vi "CENTRIOD DETECTION.vi"(0 "Refnum in":T6=refnum, 1 "auto threshold":bool, 2 "Threshold Range In":cluster{"Lower value":sgl, "Upper value":sgl}={"Lower value"=128.0, "Upper value"=255.0} {"Upper value" format="%.2f"; "Lower value" format="%.2f"}, 4 "beam detection para":T4={"Filter"=1, "Filter Para"={"X Size"=5, "Y Size"=5, "% Tolerance"=1}, "detection method"=4, "smal para"=[{"Measurement Parameter"=35, "Range Lower Value"=0.0, "Range Upper Value"=500.0, "Range"=TRUE, "Measurement Type"=FALSE}], "Remove small Objects"=TRUE, "Restrict to round Objects"=TRUE} {"smal para"."Measurement Parameter" items=["Center of Mass X", "Center of Mass Y", "First Pixel X", "First Pixel Y", "Bounding Rect Left", "Bounding Rect Top", "Bounding Rect Right", "Bounding Rect Bottom", "Max Feret Diameter Start X", "Max Feret Diameter Start Y", "Max Feret Diameter End X", "Max Feret Diameter End Y", "Max Horiz. Segment Length Left", "Max Horiz. Segment Length Right", "Max Horiz. Segment Length Row", "-", "Bounding Rect Width", "Bounding Rect Height", "Bounding Rect Diagonal", "Perimeter", "Convex Hull Perimeter", "Holes' Perimeter", "Max Feret Diameter", "Equivalent Ellipse Major Axis", "Equivalent Ellipse Minor Axis", "Equivalent Ellipse Minor Axis (Feret)", "Equivalent Rect Long Side", "Equivalent Rect Short Side", "Equivalent Rect Diagonal", "Equivalent Rect Short Side (Feret)", "Average Horiz. Segment Length", "Average Vert. Segment Length", "Hydraulic Radius", "Waddel Disk Diameter", "-", "Area", "Holes' Area", "Particle & Holes' Area", "Convex Hull Area", "Image Area", "-", "Number of Holes", "Number of Horiz. Segments", "Number of Vert. Segments", "-", "Orientation", "Max Feret Diameter Orientation", "-", "% Area/Image Area", "% Area/(Particle & Holes' Area)", "Ratio of Equivalent Ellipse Axes", "Ratio of Equivalent Rect Sides", "-", "Elongation Factor", "Compactness Factor", "Heywood Circularity Factor", "Type Factor", "-", "Sum X", "Sum Y", "Sum XX", "Sum XY", "Sum YY", "Sum XXX", "Sum XXY", "Sum XYY", "Sum YYY", "-", "Moment of Inertia XX", "Moment of Inertia XY", "Moment of Inertia YY", "Moment of Inertia XXX", "Moment of Inertia XXY", "Moment of Inertia XYY", "Moment of Inertia YYY", "Norm. Moment of Inertia XX", "Norm. Moment of Inertia XY", "Norm. Moment of Inertia YY", "Norm. Moment of Inertia XXX", "Norm. Moment of Inertia XXY", "Norm. Moment of Inertia XYY", "Norm. Moment of Inertia YYY", "Hu Moment 1", "Hu Moment 2", "Hu Moment 3", "Hu Moment 4", "Hu Moment 5", "Hu Moment 6", "Hu Moment 7"]; "smal para"."Range Lower Value" format="%.2f"; "smal para"."Range Upper Value" format="%.2f"; "detection method" items=["clustering", "entropy", "metric", "moments", "inter-class variance"]; "Filter" items=["No Filter", "Median Filter", "Low Pass Filter"]}, 5 "error in (no error)":errorcluster) -> (8 "Bounding Rect":T7={"Left"=200.0, "Top"=222.0, "Right"=337.0, "Bottom"=354.0}, 11 "Particle Reports (Pixels)":T8(array[cluster])=[{"Area"=13217.0, "Number of Holes"=0.0, "Bounding Rect"={"Left"=200.0, "Top"=222.0, "Right"=337.0, "Bottom"=354.0}, "Center of Mass"={"X"=269.13989558901415, "Y"=287.03949459030036}, "Orientation"=28.32814462161336, "Dimensions"={"Width"=137.0, "Height"=132.0}}] {"Orientation" format="%.2f"; "Dimensions"."Height" format="%.2f"; "Dimensions"."Width" format="%.2f"; "Center of Mass"."Y" format="%.2f"; "Center of Mass"."X" format="%.2f"; "Bounding Rect"."Bottom" format="%.2f"; "Bounding Rect"."Right" format="%.2f"; "Bounding Rect"."Top" format="%.2f"; "Bounding Rect"."Left" format="%.2f"; "Number of Holes" format="%.2f"; "Area" format="%.2f"}, 12 "Threshold Range Out":cluster{"Lower value":sgl, "Upper value":sgl}={"Lower value"=128.0, "Upper value"=255.0} {"Upper value" format="%.2f"; "Lower value" format="%.2f"}, 13 "Area":dbl=13217.0, 14 "Refnum out":T6, 17 "Number of Particles":i32=1, 18 "Centriod":cluster{"X":dbl, "Y":dbl}={"X"=268.53924560546875, "Y"=286.7691955566406}, 19 "error out":errorcluster)   [LabVIEW 2020]
uses:
  <vilib>/vision/Image Controls.llb/IMAQ Image.ctl
  Ctrs/beam detection.ctl
  <vilib>/vision/Measure.llb/Edge Options.ctl
  <vilib>/vision/Measure.llb/Edge Polarity.ctl
  <vilib>/vision/NI_Vision_Development_Module.lvlib
panel:
  out "Circle Found":bool=TRUE
  in  "Options":T3={"Search  Direction"=1, "Edge Options"={"Edge Polarity"=2, "Kernel Size"=3, "Width"=3, "Minimum Edge Strength"=10.0, "Interpolation Type"=enum."Bilinear Fixed", "Data Processing Method"=enum."Average"}, "Show Search Area"=FALSE, "Show Search Lines"=FALSE, "Show Edges Found"=FALSE, "Show Result"=TRUE, "Search Area Color"=65280, "Search Lines Color"=255, "Edge Locations Color"=16776960, "Result Color"=3079978, "Overlay Group Name"=""} {"Search  Direction" items=["Outside to Inside", "Inside to Outside"]; "Edge Options"."Edge Polarity" items=["All Edges", "Rising Edges", "Falling Edges"]; "Edge Options"."Minimum Edge Strength" format="%.2f"; "Edge Options"."Width" step=2; "Edge Options"."Kernel Size" step=2}
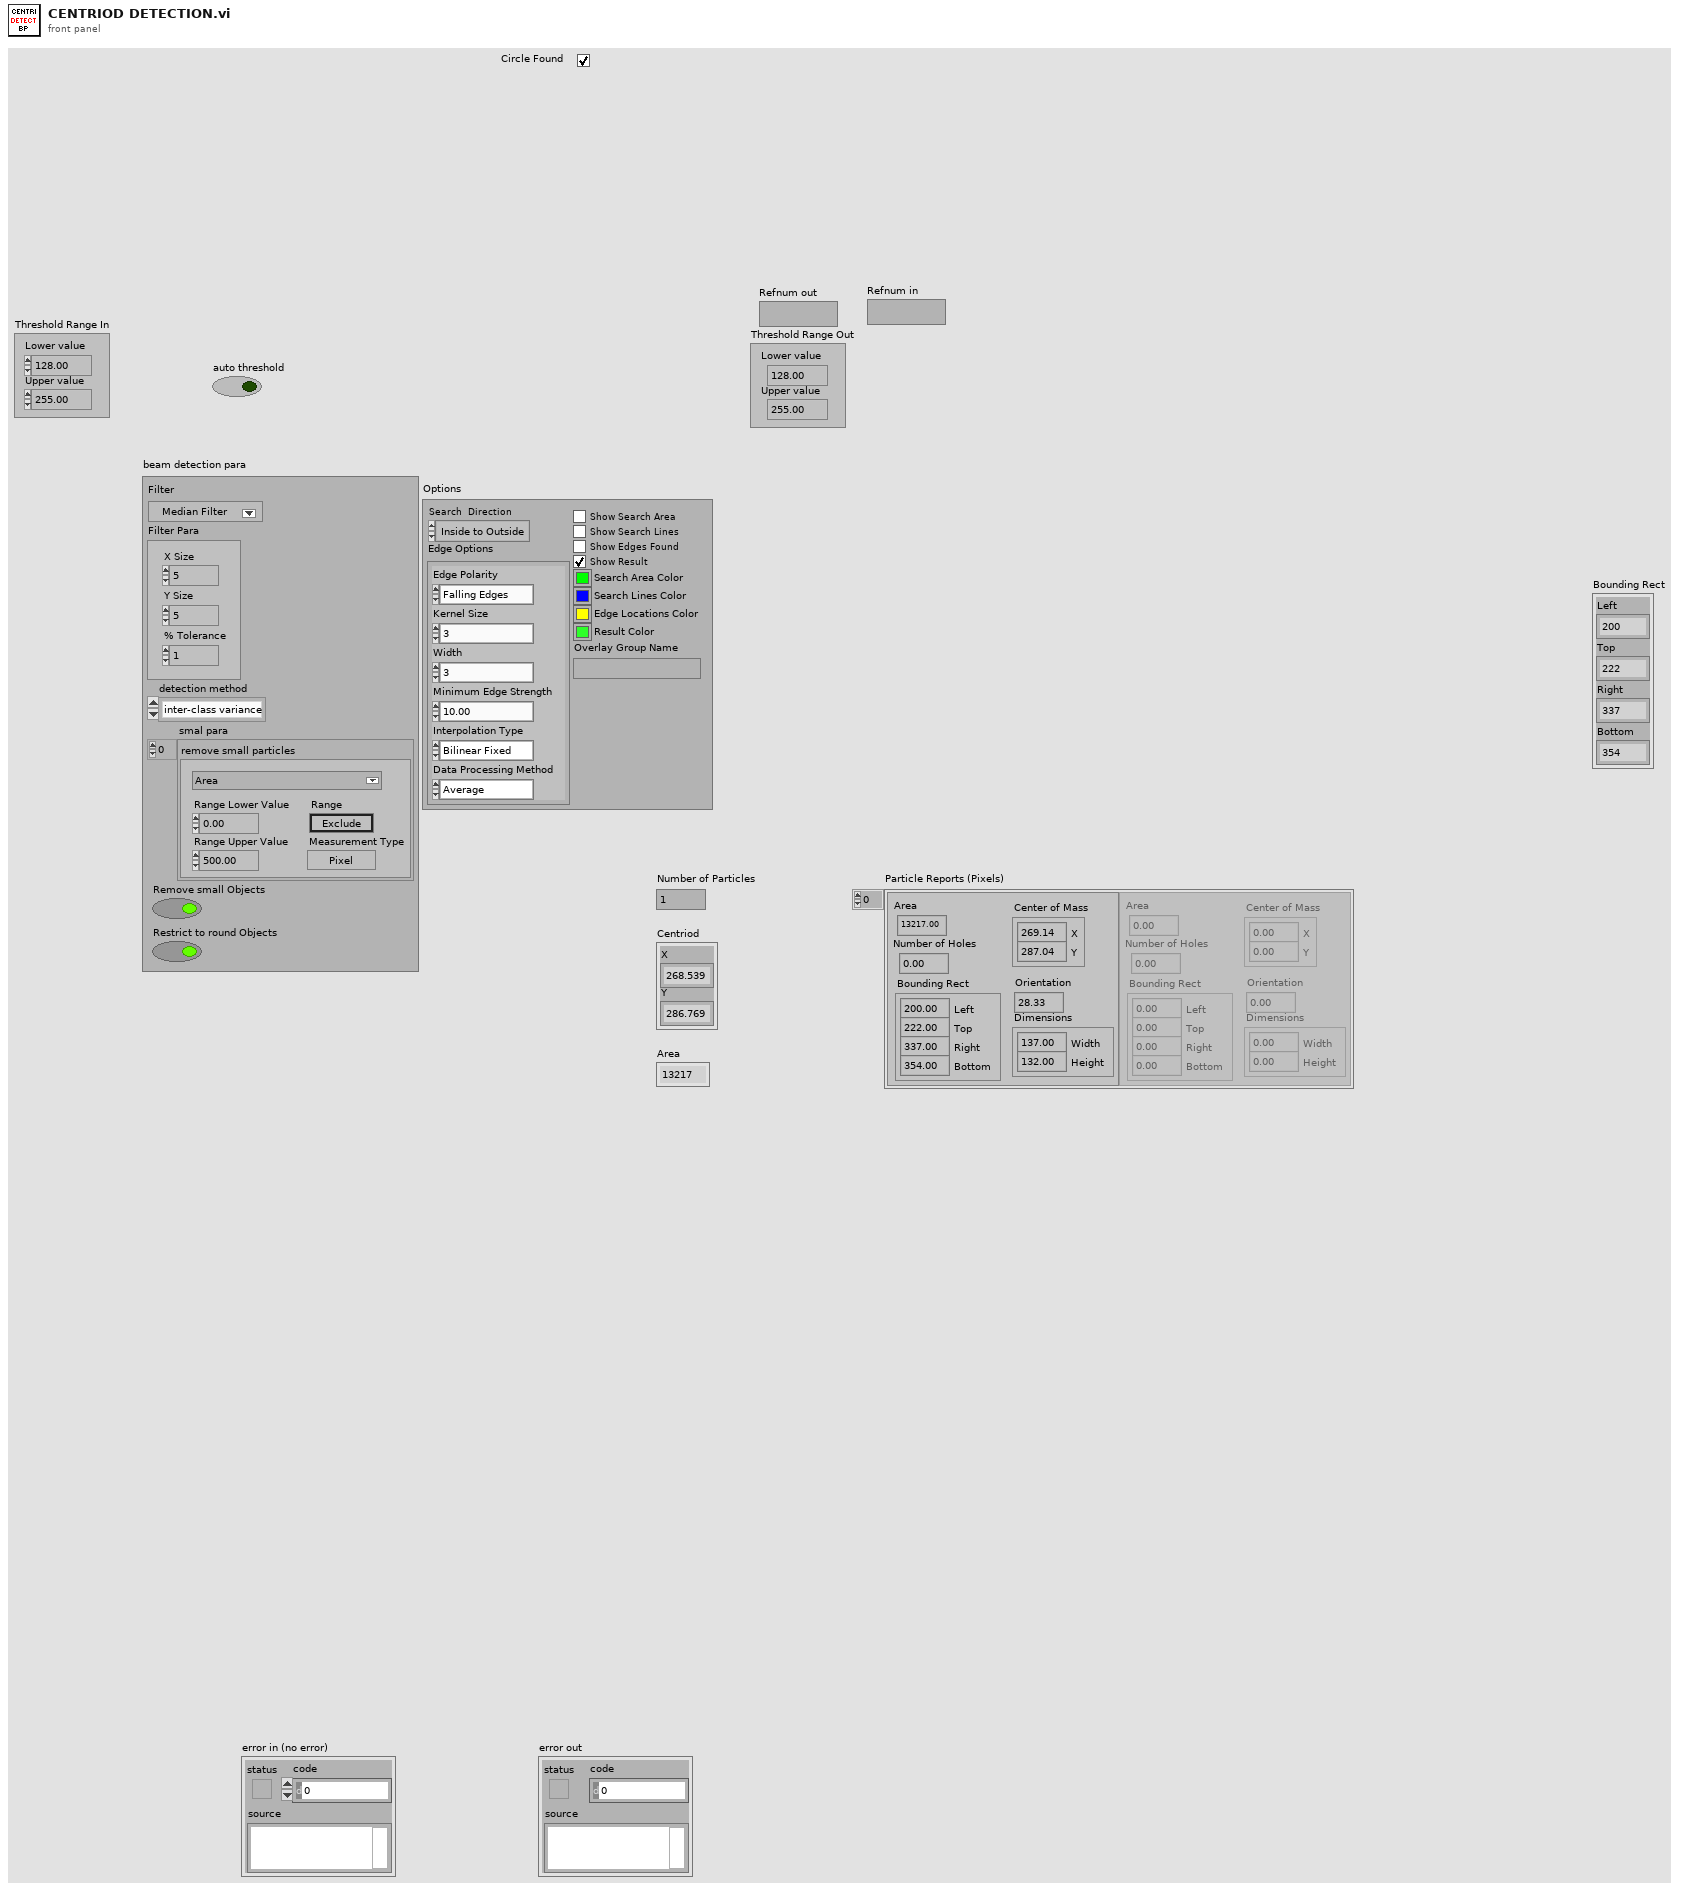
[diagram p1: front panel]
types:
  T1 = typedef "Edge Options.ctl" = cluster{"Edge Polarity":T2, "Kernel Size":u32, "Width":u32, "Minimum Edge Strength":sgl, "Interpolation Type":enum32{"Zero Order", "Bilinear", "Quadratic", "Cubic", "Bilinear Fixed"}, "Data Processing Method":enum32{"Average", "Median"}}
  T2 = typedef "Edge Polarity.ctl" = u32
  T3 = cluster{"Search  Direction":u32, "Edge Options":T1, "Show Search Area":bool, "Show Search Lines":bool, "Show Edges Found":bool, "Show Result":bool, "Search Area Color":u32, "Search Lines Color":u32, "Edge Locations Color":u32, "Result Color":u32, "Overlay Group Name":string}
  T4 = typedef "beam detection.ctl" = cluster{"Filter":u16, "Filter Para":cluster{"X Size":i32, "Y Size":i32, "% Tolerance":i32}, "detection method":i32, "smal para":cluster{"Measurement Parameter":T5, "Range Lower Value":dbl, "Range Upper Value":dbl, "Range":bool, "Measurement Type":bool}[], "Remove small Objects":bool, "Restrict to round Objects":bool}
  T5 = typedef "Particle Parameters" = i32
  T6 = typedef "IMAQ Image.ctl" = refnum<image>
  T7 = cluster{"Left":dbl, "Top":dbl, "Right":dbl, "Bottom":dbl}
  T8 = cluster{"Area":dbl, "Number of Holes":dbl, "Bounding Rect":cluster{"Left":dbl, "Top":dbl, "Right":dbl, "Bottom":dbl}, "Center of Mass":cluster{"X":dbl, "Y":dbl}, "Orientation":dbl, "Dimensions":cluster{"Width":dbl, "Height":dbl}}[]
  T9 = typedef "Image Type" = u32
  T10 = cluster{"X Size":i32, "Y Size":i32, "% Tolerance":i32}
  T11 = typedef "IMAQ Circle" = cluster{"Center X":i32, "Center Y":i32, "Inner Radius":i32, "Outer Radius":i32, "Start Angle":dbl, "End Angle":dbl}
  T12 = cluster{"Measurement Parameter":T5, "Range Lower Value":dbl, "Range Upper Value":dbl, "Range":bool, "Measurement Type":bool}[]
  T13 = cluster{"Area":dbl, "Number of Holes":dbl, "Bounding Rect":cluster{"Left":dbl, "Top":dbl, "Right":dbl, "Bottom":dbl}, "Center of Mass":cluster{"X":dbl, "Y":dbl}, "Orientation":dbl, "Dimensions":cluster{"Width":dbl, "Height":dbl}}
  T14 = typedef "ROI Descriptor" = cluster{"Global Rectangle":i32[], "Contours":cluster{"ID":enum32{"External", "Internal"}, "Type":u32, "Coordinates":i32[]}[]}
  T15 = cluster{"Center (Pixels)":cluster{"X":sgl, "Y":sgl}, "Radius (Pixels)":dbl, "Center (Real-World)":cluster{"X":sgl, "Y":sgl}, "Radius (Real-World)":dbl, "Roundness (Real-World)":dbl, "Average Strength":dbl, "Average SNR (dB)":dbl}
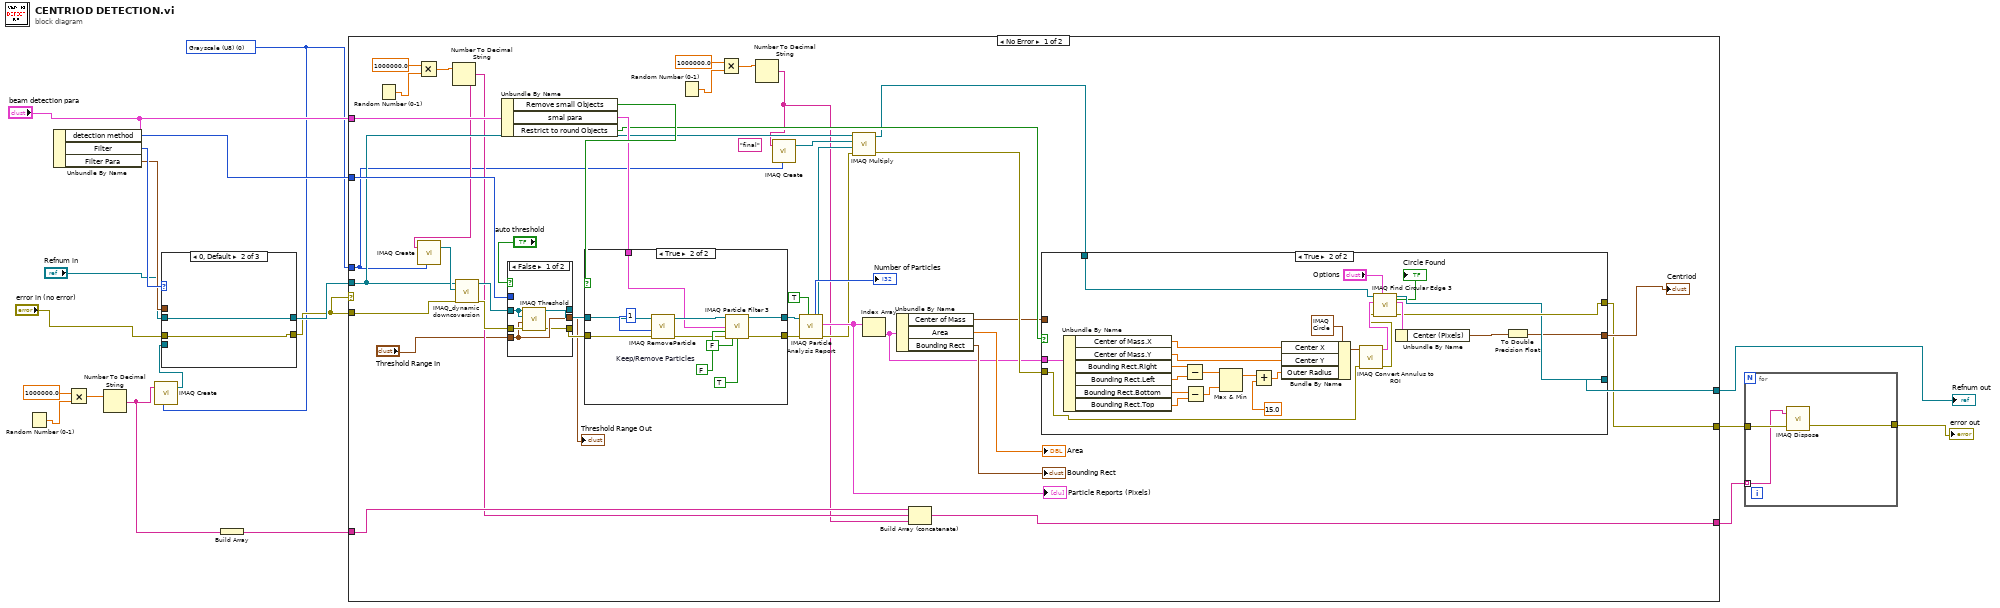
[diagram p0: block diagram]
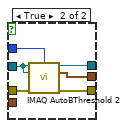
[diagram p2: hidden frame]
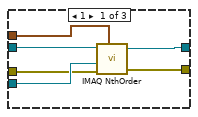
[diagram p6: hidden frame]
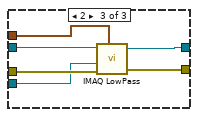
[diagram p7: hidden frame]
diagram:
  w1 = T9 0 items=["Grayscale (U8)", "Grayscale (I16)", "Grayscale (SGL)", "Complex (CSG)", "RGB (U32)", "HSL (U32)", "RGB (U64)", "Grayscale (U16)"] ("Image Type")
  n1 = Random Number (0-1)() -> (number: 0 to 1=w10:dbl)
  n2 = Unbundle By Name("beam detection para") -> ("detection method"=w17:i32, "Filter"=w18:u16, "Filter Para"=w16:T10)
  n3 = Multiply(x=1000000.0, y=w10) -> (x*y=w8:dbl)
  n4 = Number To Decimal String(number=w8) -> (decimal integer string=w6:string)  [unwired: 1 in]
  n5 = call "IMAQ Create"("Image Name"=w6, "Image Type"=w1) -> ("New Image"=w19:T6)  [unwired: 3 in, 1 out]
  n6 = case shown="0, Default" w18 {
    tunnel: "error in (no error)" -> [w22 w26 w33]
    tunnel: "Refnum in" -> [w24 w27 w28]
    tunnel: w16 -> [w25 _ w32]
    tunnel: [w20 w27 w31] -> w14
    tunnel: w19 -> [w23 _ w30]
    tunnel: [w21 w26 w29] -> w12
    frame 1 {
      n7 = call "IMAQ NthOrder"("Image Src"=w24, "Size & Order #"=w25, "Image Dst"=w23, "error in (no error)"=w22) -> ("Image Dst Out"=w20:T6, "error out"=w21:errorcluster)  [unwired: 3 in]
    }
    frame 0, Default {
    }
    frame 2 {
      n8 = call "IMAQ LowPass"("Image Src"=w28, "Size & Tolerance"=w32, "Image Dst"=w30, "error in (no error)"=w33) -> ("Image Dst Out"=w31:T6, "error out"=w29:errorcluster)  [unwired: 3 in]
    }
  }
  n9 = Build Array(w6) -> (w7:string[])
  n10 = case shown="No Error" w12 {
    tunnel: w12 -> [w75 w130]
    tunnel: w17 -> [w65 _]
    tunnel: "beam detection para" -> [w64 _]
    tunnel: w14 -> [w58 w131]
    tunnel: [w52 w131] -> w2
    tunnel: [w45 w130] -> w5
    tunnel: w7 -> [w44 w129]
    tunnel: [w42 w129] -> w4
    tunnel: w1 -> [w35 _]
    frame No Error {
      (unwired) "final" ("Image Name")
      n11 = Random Number (0-1)() -> (number: 0 to 1=w49:dbl)
      n12 = Multiply(x=1000000.0, y=w49) -> (x*y=w51:dbl)
      n13 = Number To Decimal String(number=w51) -> (decimal integer string=w43:string)  [unwired: 1 in]
      n14 = call "IMAQ Create"("Image Name"=w43, "Image Type"=w35) -> ("New Image"=w72:T6)  [unwired: 3 in, 1 out]
      n15 = call "IMAQ_dynamic downcoversion.vi"("error in (no error)"=w75, "Image Dst"=w72, "Image Src"=w58) -> ("error out"=w74:errorcluster, "Image Out"=w73:T6)  [unwired: 7 in]
      n16 = Unbundle By Name(w64) -> ("Remove small Objects"=w63:bool, "smal para"=w62:T12, "Restrict to round Objects"=w60:bool)
      n17 = case shown="False" "auto threshold" {
        tunnel: w74 -> [w81 w87]
        tunnel: w73 -> [w80 w86]
        tunnel: [w77 w85] -> w68
        tunnel: [w79 w84] -> w67
        tunnel: w65 -> [_ w83]
        tunnel: [w78 w82] -> w39
        tunnel: "Threshold Range In" -> [w78 _]
        frame False {
          n18 = call "IMAQ Threshold"("error in (no error)"=w81, "Range"=w78, "Image Dst"=w80, "Image Src"=w80) -> ("error out"=w77:errorcluster, "Image Dst Out"=w79:T6)  [unwired: 6 in]
        }
        frame True {
          n19 = call "IMAQ AutoBThreshold 2"("Image Src"=w86, "Method (clustering)"=w83, "Image Dst"=w86, "error in (no error)"=w87) -> ("Image Dst Out"=w84:T6, "Threshold Range Out"=w82:cluster{"Lower value":sgl, "Upper value":sgl}, "error out"=w85:errorcluster)  [unwired: 9 in]
        }
      }
      "Threshold Range Out" <- w39
      n20 = case shown="True" w63 {
        tunnel: [w117 w124] -> w69
        tunnel: [w116 w123] -> w70
        tunnel: w67 -> [w117 w122]
        tunnel: w68 -> [w116 w121]
        tunnel: w62 -> [_ w119]
        frame False {
        }
        frame True {
          w128 = FALSE  # Keep/Remove Particles
          n21 = call "IMAQ RemoveParticle"("error in (no error)"=w121, "Number of Erosion"=1 ("Numeric"), "Image Src"=w122) -> ("error out"=w125:errorcluster, "Image Dst Out"=w126:T6)  [unwired: 4 in, 3 out]
          n22 = call "IMAQ Particle Filter 3"("Image Src"=w126, "Selection Values"=w119, "Keep/Remove Particles (F)"=w128, "error in (no error)"=w125, "Reject Border? (F)"=FALSE, "Fill Holes? (F)"=TRUE) -> ("Image Dst Out"=w124:T6, "error out"=w123:errorcluster)  [unwired: 3 in, 5 out]
        }
      }
      n23 = Random Number (0-1)() -> (number: 0 to 1=w48:dbl)
      n24 = Multiply(x=1000000.0, y=w48) -> (x*y=w46:dbl)
      n25 = Number To Decimal String(number=w46) -> (decimal integer string=w36:string)  [unwired: 1 in]
      n26 = call "IMAQ Create"("Image Name"=w36, "Image Type"=w35) -> ("New Image"=w71:T6)  [unwired: 3 in, 1 out]
      n27 = call "IMAQ Particle Analysis Report"("Connectivity 4/8 (8)"=TRUE, "error in (no error)"=w70, "Image"=w69) -> ("error out"=w40:errorcluster, "Particle Reports (Pixels)"=w57:T8, "Image Out (duplicate)"=w41:T6, "Number of Particles"=→"Number of Particles":i32)  [unwired: 3 in, 2 out]
      "Particle Reports (Pixels)" <- w57
      n28 = call "IMAQ Multiply"("Image Src A"=w58, "Image Dst"=w71, "Image Src B"=w41, "error in (no error)"=w40) -> ("Image Dst Out"=w55:T6, "error out"=w59:errorcluster)  [unwired: 3 in]
      n29 = Index Array(array=w57) -> (element=w56:T13)  [unwired: 1 in]
      n30 = Unbundle By Name(w56) -> ("Center of Mass"=w54:cluster{"X":dbl, "Y":dbl}, "Area"=→"Area":dbl, "Bounding Rect"=→"Bounding Rect":T7)
      n31 = Build Array (concatenate)(w44, w43, w36) -> (w42:string[])
      n32 = case shown="True" w60 {
        tunnel: w55 -> [w88 w115]
        tunnel: [w90 w108] -> w53
        tunnel: w54 -> [w90 _]
        tunnel: w59 -> [w89 w102]
        tunnel: [w89 w112] -> w45
        tunnel: [w88 w111] -> w52
        tunnel: w56 -> [_ w105]
        frame False {
        }
        frame True {
          n33 = Unbundle By Name(w105) -> ("Center of Mass.X"=w92:dbl, "Center of Mass.Y"=w91:dbl, "Bounding Rect.Right"=w97:dbl, "Bounding Rect.Left"=w96:dbl, "Bounding Rect.Bottom"=w95:dbl, "Bounding Rect.Top"=w94:dbl)
          n34 = Subtract(x=w97, y=w96) -> (x-y=w98:dbl)
          n35 = Subtract(x=w95, y=w94) -> (x-y=w99:dbl)
          n36 = Max & Min(x=w98, y=w99) -> (max(x,y)=w100:dbl)  [unwired: 1 out]
          n37 = Add(x=w100, y=15.0) -> (x+y=w93:dbl)
          n38 = Bundle By Name(cluster=T11 {"Center X"=0, "Center Y"=0, "Inner Radius"=0, "Outer Radius"=0, "Start Angle"=0.0, "End Angle"=360.0} ("Annulus"), "Center X"=w92, "Center Y"=w91, "Outer Radius"=w93) -> (w106:T11)
          n39 = call "IMAQ Convert Annulus to ROI"("error in (no error)"=w102, "Annulus"=w106) -> ("error out"=w103:errorcluster, "ROI Descriptor"=w104:T14)  [unwired: 7 in]
          n40 = call "IMAQ Find Circular Edge 3"("Options"="Options", "error in (no error)"=w103, "ROI Descriptor"=w104, "Image"=w115) -> ("error out"=w112:errorcluster, "Fitted Circle"=w113:T15, "Image Out"=w111:T6, "Circle Found"=→"Circle Found":bool)  [unwired: 3 in, 1 out]
          n41 = Unbundle By Name(w113) -> ("Center (Pixels)"=w109:cluster{"X":sgl, "Y":sgl})
          n42 = To Double Precision Float(number=w109) -> (double precision float=w108:cluster{"X":dbl, "Y":dbl})
        }
      }
      "Centriod" <- w53
    }
    frame Error {
    }
  }
  "Refnum out" <- w2
  n43 = for {
    tunnel: w5 -> [w134]
    tunnel: w4 -> [w133] mode=indexing
    tunnel: [w132] -> w3
    n44 = call "IMAQ Dispose"("Image"=w133, "error in (no error)"=w134) -> ("error out"=w132:errorcluster)  [unwired: 4 in]
  }
  "error out" <- w3
